vi "Jet2_GUI.vi"(10 "stop 2":refnum<vi>, 11 "GUI_cluster":T1={"Sub Panel"=refnum, "GUIdevice"="Bella_LP_Mode", "CtlRef"=refnum, "User Event in"=refnum}) -> ()   [LabVIEW 2020]
uses:
  Shared/GUI_Template/GUI_master/tcp new data cluster.ctl
  Controls/eventtypdef1.ctl
  Shared/GUI_Template/GUI_master/tcp_new_data_event.ctl
  Controls/GUI_cluster.ctl
panel:
  in  "Link.com2::1":string caption="Jet Trigger status"
  in  "Tab Control":enum32{"Hi P Cntlr", "Med P Cntlr"}(tab)
  in  "set pressure::3":dbl caption="Hi Press. Set" min=0.0 max=600.0 format="%.1f"
  in  "read pressure::3":dbl caption="Hi Press. Read" min=0.0 max=0.0 format="%.1f"
  in  "set pressure::9":dbl caption="Med. Press. Set" min=0.0 max=150.0 format="%.1f"
  in  "read pressure::9":dbl caption="Med. Press. Read" min=0.0 max=0.0 format="%.1f"
  in  "Save::2":bool caption="Save"
  in  "trigger::2":bool caption="Trig"
  out "AI_array.Channel 0::2":waveform(dbl)[](graph) caption="Jet Voltage trace"
  in  "reading.var 28::4":dbl caption="SAC3 Convec" min=-100000.0 max=100000.0 format="%#_6e"
  in  "Delay.Ch C::5":dbl=0.042 caption="Jet Delay [s]" min=-0.1 max=0.1 format="%.5f"
  in  "reading.var 4::4":dbl caption="SAC3 Ion" min=-100000.0 max=100000.0 format="%_4e"
  in  "DigitalOutput.Channel 2::2":bool caption="Exhaust Valve"
  in  "Jet Trigger":bool caption="Jet Trig"
  out "GUIdevice 1":string="StagingNISwitch"
  out "GUIdevice 2":string="Staging_USB6210_1"
  out "GUIdevice 3":string="StagingHighPressureController"
  out "GUIdevice 4":string="DS-A-Cave_VacSys_Feedback_Double"
  out "GUIdevice 5":string="StagingDG645_2"
  out "GUIdevice 6":string="StagingLowPressure1"
  out "GUIdevice 7":string="StagingDischargeHV"
  out "GUIdevice 8":string="StagingLowPressure2"
  out "GUIdevice 9":string="StagingMedPController"
  in  "stop":bool
  out "tcp data event":T2
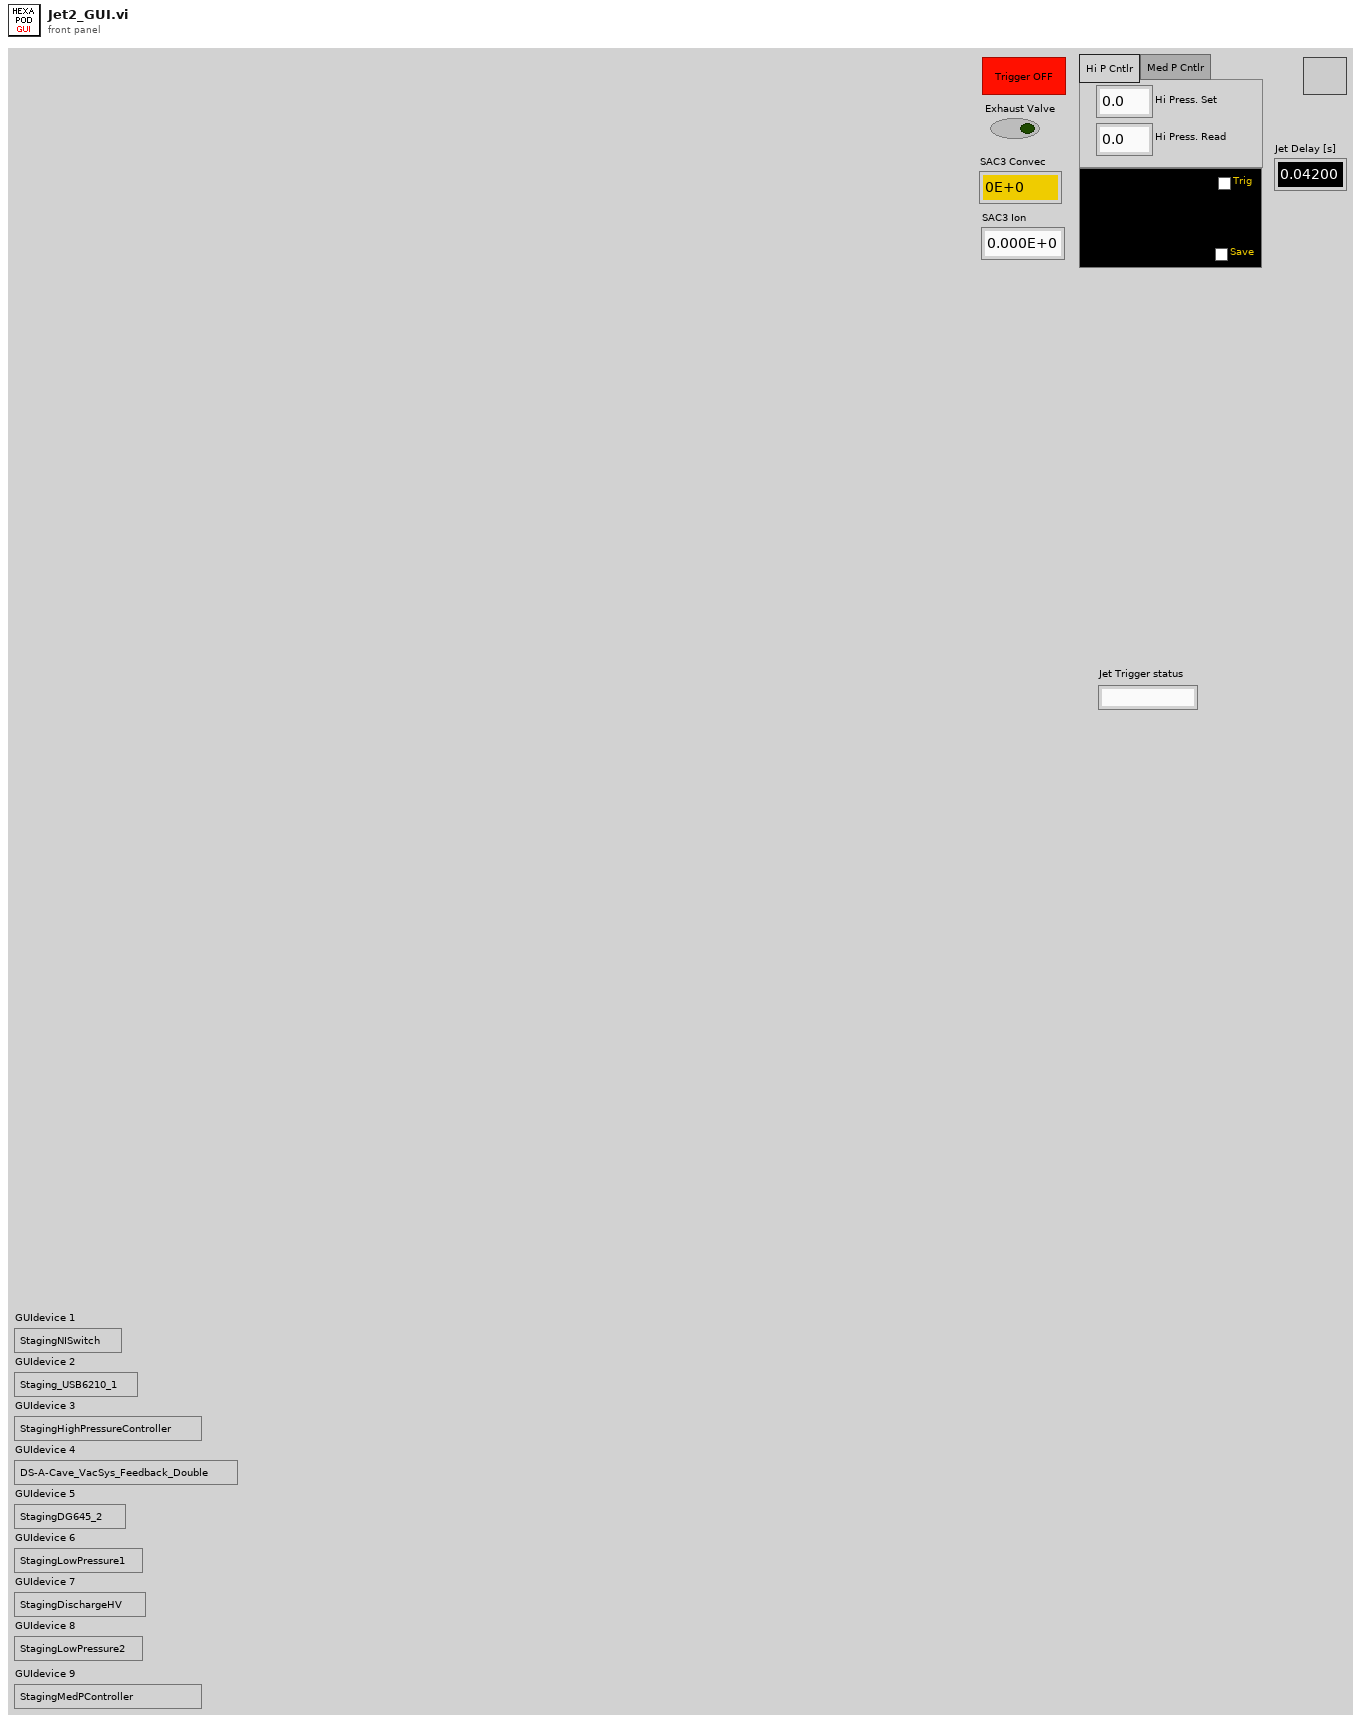
[diagram p1: front panel]
types:
  T1 = typedef "GUI_cluster.ctl" = cluster{"Sub Panel":refnum<vi>, "GUIdevice":string, "CtlRef":refnum<vi>, "User Event in":refnum<user-event>}
  T2 = typedef "tcp_new_data_event.ctl" = refnum<user-event>
  T3 = typedef "eventtypdef1.ctl" = cluster{"label":string, "Sub Panel":refnum<vi>, "CtlRef":refnum<vi>, "This VI":refnum<vi>}
  T4 = typedef "tcp new data cluster.ctl" = cluster{"EventEnum":enum16{"new data", "connection status update"}, "Device name":string}
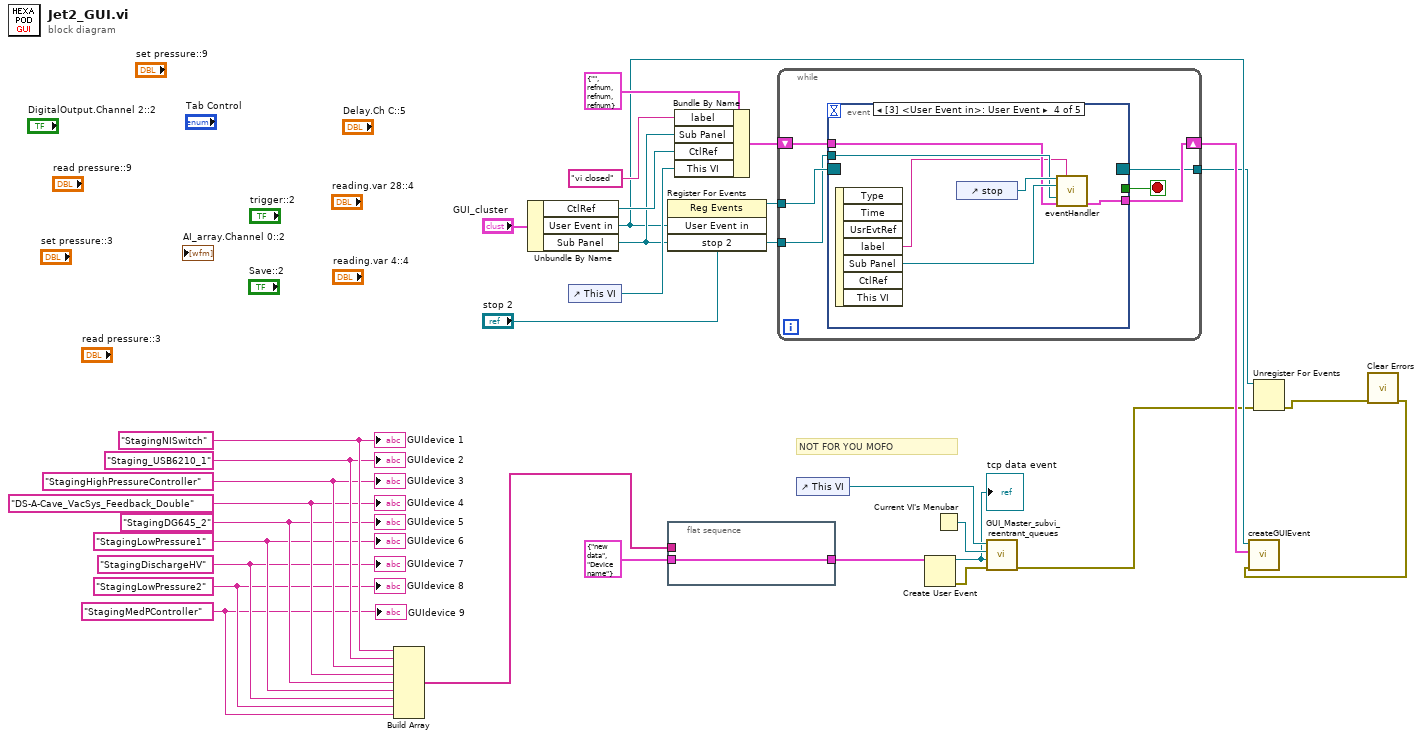
[diagram p0: block diagram]
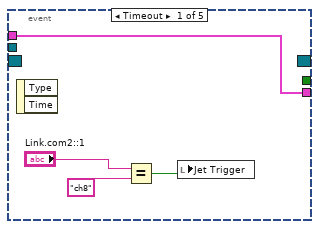
[diagram p2: hidden frame]
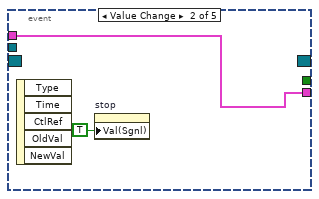
[diagram p3: hidden frame]
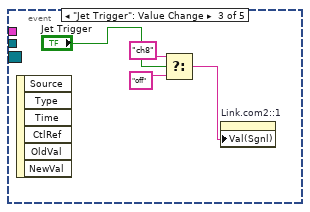
[diagram p4: hidden frame]
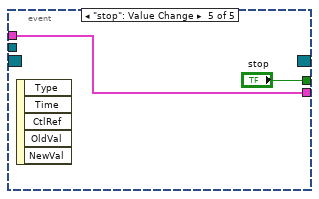
[diagram p5: hidden frame]
diagram:
  w2 = "StagingMedPController" ("GUIdevice 6")
  w3 = "StagingLowPressure2" ("GUIdevice 6")
  w4 = "StagingDischargeHV" ("GUIdevice 23")
  w5 = "StagingLowPressure1" ("GUIdevice 6")
  w6 = "StagingDG645_2" ("GUIdevice 5")
  w7 = "DS-A-Cave_VacSys_Feedback_Double" ("GUIdevice 4")
  w8 = "StagingHighPressureController" ("GUIdevice 3")
  w9 = "Staging_USB6210_1" ("GUIdevice 2")
  w10 = "StagingNISwitch" ("GUIdevice 1")
  # "NOT FOR YOU MOFO"
  n1 = Build Array(w10, w9, w8, w7, w6, w5, w4, w3, w2) -> (w1:string[])
  n2 = Unbundle By Name("GUI_cluster") -> ("CtlRef"=w23:refnum<vi>, "User Event in"=w17:refnum<user-event>, "Sub Panel"=w19:refnum<vi>)
  n3 = control-ref of="This VI"() -> (w22:refnum<vi>)
  n4 = register-events(w17, "stop 2") -> (reference out=w21:refnum<event-registration>)  [unwired: 2 in, 1 out]
  n5 = flat-sequence {
    tunnel: T4 {"EventEnum"=enum."new data", "Device name"="Device name"} ("New Event") -> [w32]
    tunnel: [w32] -> w24
    tunnel: w1 -> [_]
    frame #0 {
    }
  }
  n6 = Bundle By Name(cluster=T3 {"label"="", "Sub Panel"=refnum, "CtlRef"=refnum, "This VI"=refnum} ("event data"), "label"="vi closed", "Sub Panel"=w19, "CtlRef"=w23, "This VI"=w22) -> (w18:T3)
  n7 = while {
    tunnel: w21 -> [w38]
    tunnel: w19 -> [w36]
    shift-right: [w34] -> w16
    shift-left: w18 -> [w35]
    tunnel: [w33] -> w13
    stop <- w37 stop-if-true
    n8 = event shown="[3] <User Event in>: User Event" {
      selector: w38 -> [_ _ _ _ _]
      dyn-events: [_ _ _ _ _] -> w33
      timeout: _ -> [_ _ _ _ _]
      tunnel: [_ _ _ _ "stop"] -> w37
      tunnel: w36 -> [_ _ _ w52 _]
      tunnel: w35 -> [w42 w44 _ w51 w55]
      tunnel: [w42 w44 _ w50 w55] -> w34
      event Timeout {
        n9 = event-data() -> ()  [unwired: 1 in, 2 out]
        n10 = Equal?(x="Link.com2::1", y="ch8") -> (x = y?=w40:bool)
        n11 = local write "Jet Trigger"(w40) -> ()
      }
      event Value Change {
        n12 = event-data() -> ()  [unwired: 1 in, 5 out]
        n13 = property on="stop" class="Bool (strict)"("Val(Sgnl)"=TRUE ("Value (Signaling)")) -> ()  [unwired: 2 in, 2 out]
      }
      event "Jet Trigger": Value Change {
        n14 = event-data() -> ()  [unwired: 1 in, 6 out]
        n15 = Select(t="ch8", s="Jet Trigger", f="off") -> (s? t:f=w45:string)
        n16 = property on="Link.com2::1" class="Str"("Val(Sgnl)"=w45) -> ()  [unwired: 2 in, 2 out]
      }
      event User Event {
        n17 = event-data() -> ("label"=w49:string, "Sub Panel"=w53:refnum<vi>)  [unwired: 1 in, 5 out]
        n18 = control-ref of="stop"() -> (w54:refnum<vi>)
        n19 = call "eventHandler.vi"("Boolean in"=w54, "label"=w49, "Sub Panel 2"=w53, "Sub Panel"=w52, "event data in"=w51) -> ("event data out"=w50:T3)  [unwired: 10 in]
      }
      event "stop": Value Change {
        n20 = event-data() -> ()  [unwired: 1 in, 5 out]
      }
    }
  }
  n21 = control-ref of="This VI"() -> (w31:refnum<vi>)
  n22 = Create User Event(user event datatype=w24) -> (user event=w28:refnum<user-event>, error out=w29:errorcluster)  [unwired: 1 in]
  "tcp data event" <- w28
  n23 = Current VI's Menubar() -> (w30:refnum<k9>)
  n24 = call "GUI_Master_subvi_reentrant_queues.vi"("error in (no error)"=w29, "tcp data event"=w28, "Caller menu reference"=w30, "Caller VI ref"=w31) -> ("error out"=w12:errorcluster)  [unwired: 7 in]
  n25 = Unregister For Events(event registration refnum=w13, error in=w12) -> (error out=w14:errorcluster)
  n26 = call <vilib>:"Clear Errors.vi"("error in (no error)"=w14) -> ("error out"=w11:errorcluster)  [unwired: 5 in, 1 out]
  n27 = call "createGUIEvent.vi"("error in (no error)"=w11, "event data"=w16, "User Event in"=w17) -> ()  [unwired: 8 in, 1 out]
  "GUIdevice 1" <- w10
  "GUIdevice 2" <- w9
  "GUIdevice 3" <- w8
  "GUIdevice 4" <- w7
  "GUIdevice 5" <- w6
  "GUIdevice 6" <- w5
  "GUIdevice 7" <- w4
  "GUIdevice 8" <- w3
  "GUIdevice 9" <- w2
